vi "main 01.vi"() -> ()   [LabVIEW 2018]
uses:
  Global Value.vi
panel:
  out "상태":string
  in  "종료":bool
  in  "접속":bool
  out "CommConnect":i32
  in  "KHOpenAPI":refnum<k7>(container)
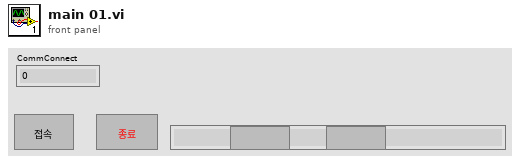
[diagram p1: front panel]
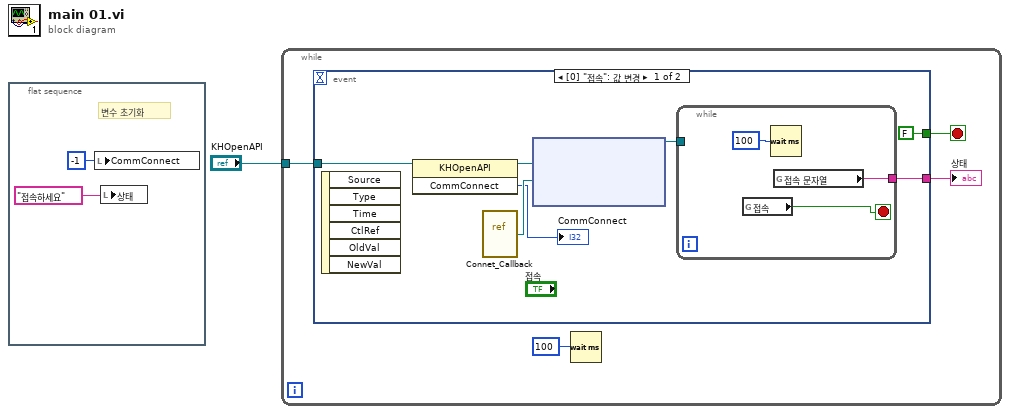
[diagram p0: block diagram]
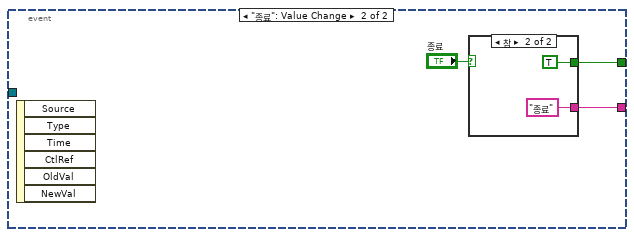
[diagram p2: hidden frame]
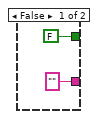
[diagram p3: hidden frame]
diagram:
  n1 = flat-sequence {
    frame #0 {
      # "변수 초기화"
      n2 = local write "CommConnect"(-1 ("CommConnect")) -> ()
      n3 = local write "상태"("접속하세요" ("상태")) -> ()
    }
  }
  n4 = while {
    tunnel: "KHOpenAPI" -> [w5]
    stop <- w6 stop-if-true
    n5 = event shown="[0] \"접속\": 값 변경" {
      selector: _ -> [_ _]
      dyn-events: _ -> [_ _]
      timeout: _ -> [_ _]
      tunnel: [w11 w19] -> w7
      tunnel: [FALSE w18] -> w6
      tunnel: w5 -> [w10 _]
      event "접속": Value Change {
        n6 = event-data() -> ()  [unwired: 1 in, 6 out]
        n7 = invoke on="인보크 노드" class="KHOpenAPI" method="CommConnect"(reference=w10) -> (reference out=w14:refnum<k7>, "CommConnect"=→"CommConnect":i32)  [unwired: 2 in, 1 out]
        n8 = vi-ref "Connet_Callback.vi"() -> ("vi reference"=w13:refnum<vi>)
        n9 = node(w14, w13) -> (w12:refnum<k27>)  [unwired: 3 in, 1 out]
        n10 = while {
          tunnel: w12 -> [_]
          tunnel: [w16] -> w11
          stop <- w15 stop-if-true
          n11 = global read "Global Value.vi" "접속"() -> (w15:bool)
          n12 = Wait (ms)(milliseconds to wait=u32 100 ("대기 시간 (ms)")) -> ()  [unwired: 1 out]
          n13 = global read "Global Value.vi" "접속 문자열"() -> (w16:string)
        }
      }
      event "종료": Value Change {
        n14 = event-data() -> ()  [unwired: 1 in, 6 out]
        n15 = case shown="참" "종료" {
          tunnel: ["" "종료"] -> w19
          tunnel: [FALSE TRUE] -> w18
          frame False {
          }
          frame True {
          }
        }
      }
    }
    "상태" <- w7
    n16 = Wait (ms)(milliseconds to wait=u32 100 ("대기 시간(ms)")) -> ()  [unwired: 1 out]
  }
